vi "Fabry-Peort-dn_change_calc.vi"(6 "dLam chnage":dbl=0.001 format="%_6g", 9 "Wavelength":dbl=1.21 format="%_6g", 10 "Et thickness at 300K":dbl=210.0 format="%.1f", 11 "Et T(K)  initial":dbl=56.5) -> (2 "Order":dbl=30.25551322702913 format="%.1f", 3 "Et T(K)  to":dbl=56.5, 4 "Temperature orders Et1 2":dbl[](array[numeric])=[30.0, 79.0289488656166, 110.46550450061054, 134.59725313809946, 155.53515021929462] format="%.2f", 5 "T and dn arr":dbl[][](array[numeric]) format="%.4f", 7 "dV(km/s) change":dbl format="%_6g")   [LabVIEW 2012]
uses:
  <vilib>/gmath/NI_Gmath.lvlib
panel:
  out "dV per order":dbl=30.25551322702913 format="%.1f"
  out "2dn at 'to' T":dbl=30.25551322702913 format="%.1f"
  out "2dn at current T":dbl=30.25551322702913 format="%.1f"
  in  "Angle to (deg)":dbl=5.0 format="%.3f"
  in  "Angle curr (deg)":dbl=5.0 format="%.3f"
  out "etalon (2dn) product  vs T(K)":cluster{"T  for integral CTE":dbl[], dbl[]}[](graph)
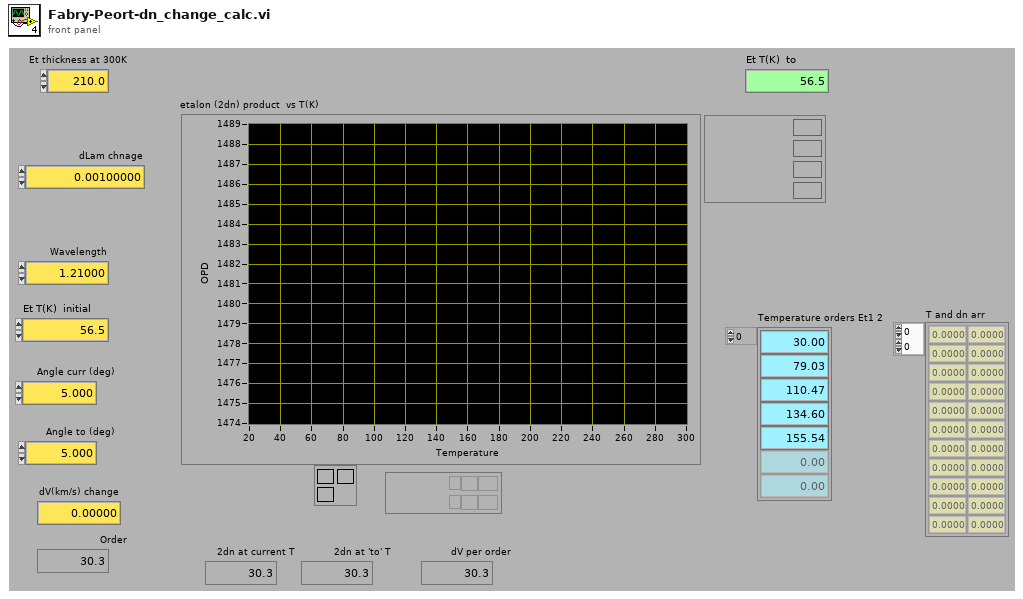
[diagram p1: front panel]
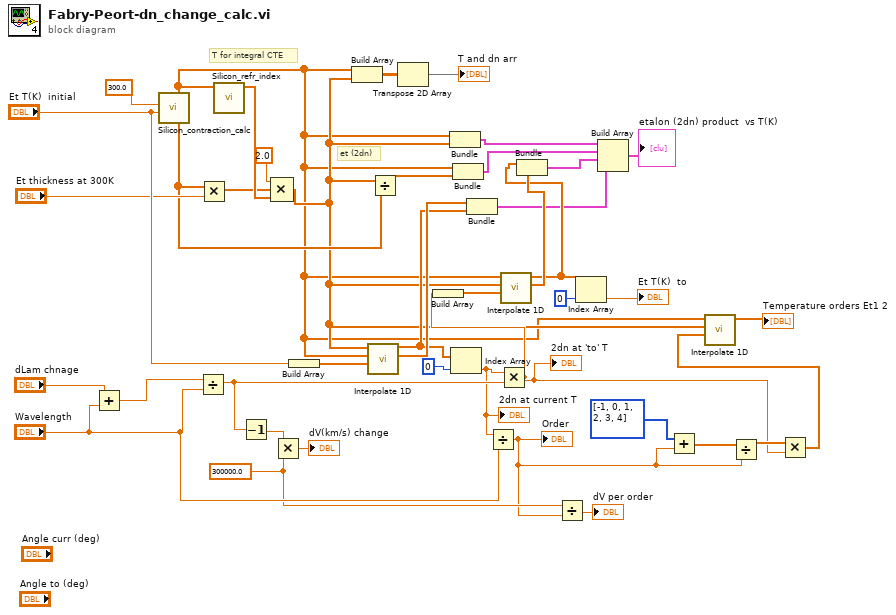
[diagram p0: block diagram]
diagram:
  w7 = 300000.0 ("y")
  # "et (2dn)"
  # "T for integral CTE"
  n1 = Add(x="dLam chnage", y="Wavelength") -> (x+y=w28:dbl)
  n2 = call "Silicon_contraction_calc.vi"("T2"="Et T(K)  initial", "T1"=300.0) -> ("Integral CTE from 300K to T"=w19:dbl[], "T  for integral CTE"=w3:dbl[])  [unwired: 4 in, 4 out]
  n3 = Divide(x=w28, y="Wavelength") -> (x/y=w18:dbl)
  n4 = Multiply(x=w19, y="Et thickness at 300K") -> (x*y=w30:dbl[])
  n5 = call "Silicon_refr_index.vi"("Temperature"=w3) -> ("Silicon refr index at T"=w38:dbl[])  [unwired: 8 in, 2 out]
  n6 = Decrement(x=w18) -> (x-1=w17:dbl)
  n7 = Compound Arithmetic op=MULTIPLY(2.0 ("value"), w30, w38) -> (w4:dbl[])
  n8 = Multiply(x=w17, y=w7) -> (x*y=→"dV(km/s) change":dbl)
  n9 = Build Array("Et T(K)  initial") -> (w35:dbl[])
  n10 = Build Array(w3, w4) -> (w2:dbl[][])
  n11 = call <vilib>:"Interpolate 1D.vi"("xi"=w35, "X"=w3, "Y"=w4) -> ("xi used"=w26:dbl[], "yi"=w21:dbl[])  [unwired: 6 in, 1 out]
  n12 = Divide(x=w4, y=w19) -> (x/y=w20:dbl[])
  n13 = Transpose 2D Array(2D array=w2) -> (transposed array=→"T and dn arr":dbl[][])
  n14 = Bundle("T  for integral CTE"=w3, w4) -> (w41:cluster{"T  for integral CTE":dbl[], dbl[]})  [unwired: 1 in]
  n15 = Index Array(array=w21, index=0) -> (element=w11:dbl)
  "2dn at current T" <- w11
  n16 = Bundle("T  for integral CTE"=w3, w20) -> (w40:cluster{"T  for integral CTE":dbl[], dbl[]})  [unwired: 1 in]
  n17 = Bundle("xi used"=w26, "yi"=w21) -> (w22:cluster{"xi used":dbl[], "yi":dbl[]})  [unwired: 1 in]
  n18 = Divide(x=w11, y="Wavelength") -> (x/y=w6:dbl)
  "Order" <- w6
  n19 = Multiply(x=w11, y=w18) -> (x*y=w10:dbl)
  "2dn at 'to' T" <- w10
  n20 = Build Array(w10) -> (w23:dbl[])
  n21 = call <vilib>:"Interpolate 1D.vi"("xi"=w23, "X"=w4, "Y"=w3) -> ("xi used"=w27:dbl[], "yi"=w25:dbl[])  [unwired: 6 in, 1 out]
  n22 = Bundle("yi"=w25, "xi used"=w27) -> (w32:cluster{"yi":dbl[], "xi used":dbl[]})  [unwired: 1 in]
  n23 = Divide(x=w7, y=w6) -> (x/y=→"dV per order":dbl)
  n24 = Index Array(array=w25, index=0) -> (element=→"Et T(K)  to":dbl)
  n25 = Build Array(w41, w40, w32, w22) -> (→"etalon (2dn) product  vs T(K)":cluster{"xi used":dbl[], "yi":dbl[]}[])
  n26 = Add(x=i32[] [-1, 0, 1, 2, 3, 4], y=w6) -> (x+y=w13:dbl[])
  n27 = Divide(x=w13, y=w6) -> (x/y=w12:dbl[])
  n28 = Multiply(x=w12, y=w10) -> (x*y=w9:dbl[])
  n29 = call <vilib>:"Interpolate 1D.vi"("xi"=w9, "X"=w4, "Y"=w3) -> ("yi"=→"Temperature orders Et1 2":dbl[])  [unwired: 6 in, 2 out]
